vi "HandleServers.vi"(8 "error in (no error)":errorcluster, 11 "S4GUI in":refnum<class "S4GUI.lvclass">) -> (0 "error out":errorcluster, 3 "S4GUI out":refnum<class "S4GUI.lvclass">)   [LabVIEW 2018, in "S4GUI.lvclass"]
uses:
  S4GUI.lvclass
  S4GUI.lvclass/S4GUI.ctl
  Server/Server.lvclass/Server.ctl
  SyncBox/Sync Box.lvclass
  C:/Users/devstaff/sparc4/s4gui/Versao ZeroMQ REQ-REP/SPARC4_GUI -v1.0.8 - reconhecimento do ACK do ACS/Server/Server.lvclass
  Instrument/Instrument.lvclass
  TCS/TCS.lvclass
  Acquisition/Acquisition.lvclass
  TelFocus/TelFocus.lvclass
  WeatherStation/WeatherStation.lvclass
  GSserver/GSserver.lvclass
  Server/Server.lvclass
panel:
  out "resto (0-3)":u32
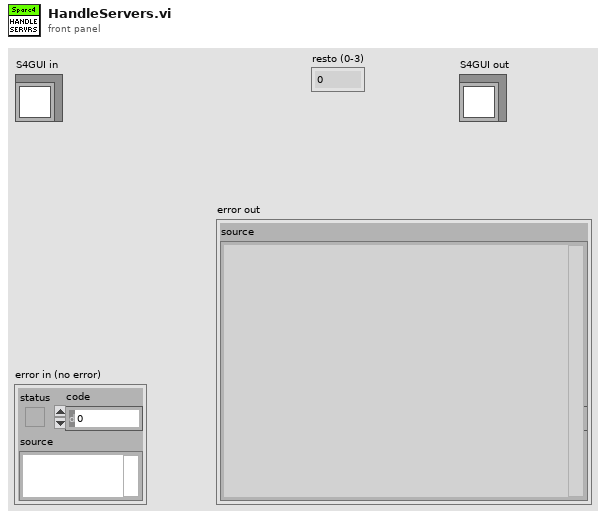
[diagram p1: front panel]
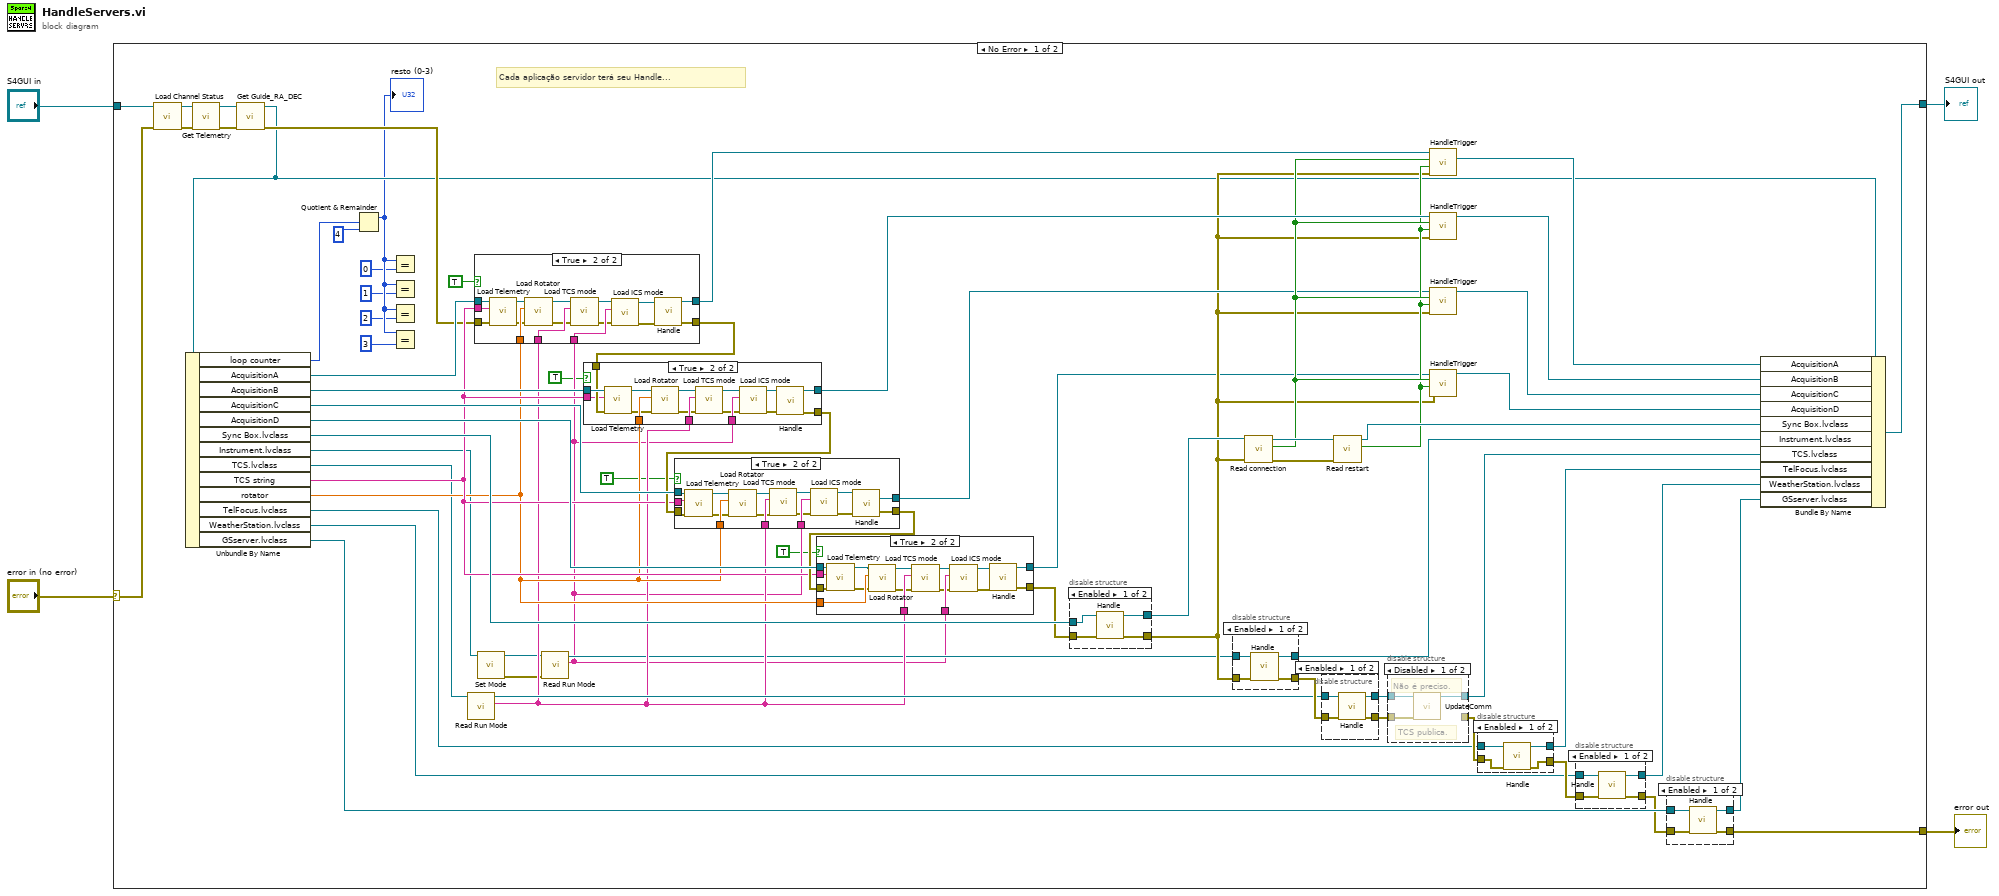
[diagram p0: block diagram]
diagram:
  n1 = case shown="No Error" "error in (no error)" {
    selector: "error in (no error)" -> [w14 w188]
    tunnel: [w5 w188] -> w3
    tunnel: [w73 w187] -> w1
    tunnel: "S4GUI in" -> [w12 w187]
    frame No Error {
      # "Cada aplicação servidor terá seu Handle..."
      n2 = call-dynamic "Load Channel Status.vi"("error in (no error)"=w14, "S4GUI in"=w12) -> ("error out"=w13:errorcluster, "S4GUI out"=w11:refnum<class "S4GUI.lvclass">)  [unwired: 8 in]
      n3 = call-dynamic "Get Telemetry.vi"("error in (no error)"=w13, "S4GUI in"=w11) -> ("error out"=w32:errorcluster, "S4GUI out"=w33:refnum<class "S4GUI.lvclass">)  [unwired: 8 in]
      n4 = call-dynamic "Get Guide_RA_DEC.vi"("error in (no error)"=w32, "S4GUI in"=w33) -> ("error out"=w31:errorcluster, "S4GUI out"=w30:refnum<class "S4GUI.lvclass">)  [unwired: 8 in]
      n5 = Unbundle By Name(w30) -> ("loop counter"=w10:u32, "AcquisitionA"=w61:refnum<class "Acquisition.lvclass">, "AcquisitionB"=w60:refnum<class "Acquisition.lvclass">, "AcquisitionC"=w58:refnum<class "Acquisition.lvclass">, "AcquisitionD"=w57:refnum<class "Acquisition.lvclass">, "Sync Box.lvclass"=w72:refnum<class "Sync Box.lvclass">, "Instrument.lvclass"=w39:refnum<class "Instrument.lvclass">, "TCS.lvclass"=w42:refnum<class "TCS.lvclass">, "TCS string"=w45:string, "rotator"=w43:dbl, "TelFocus.lvclass"=w18:refnum<class "TelFocus.lvclass">, "WeatherStation.lvclass"=w9:refnum<class "WeatherStation.lvclass">, "GSserver.lvclass"=w8:refnum<class "GSserver.lvclass">)
      n6 = Quotient & Remainder(x=w10, y=u32 4) -> (x-y*floor(x/y)=w28:u32)  [unwired: 1 out]
      "resto (0-3)" <- w28
      n7 = Equal?(x=w28, y=u32 0) -> ()  [unwired: 1 out]
      n8 = Equal?(x=w28, y=u32 1) -> ()  [unwired: 1 out]
      n9 = Equal?(x=w28, y=u32 2) -> ()  [unwired: 1 out]
      n10 = Equal?(x=w28, y=u32 3) -> ()  [unwired: 1 out]
      n11 = call-dynamic "Read Run Mode.vi"("Server in"=w42) -> ("Run mode"=w40:string, "Server out"=w41:refnum<class "TCS.lvclass">)  [unwired: 8 in, 1 out]
      n12 = call-dynamic "Set Mode.vi"("Instrument in"=w39) -> ("error out"=w37:errorcluster, "Instrument out"=w38:refnum<class "Instrument.lvclass">)  [unwired: 9 in]
      n13 = call-dynamic "Read Run Mode.vi"("error in (no error)"=w37, "Server in"=w38) -> ("Run mode"=w35:string, "Server out"=w36:refnum<class "Instrument.lvclass">)  [unwired: 7 in, 1 out]
      n14 = case shown="True" TRUE {
        tunnel: [w159 w175] -> w67
        tunnel: w61 -> [w159 w174]
        tunnel: [w158 w173] -> w59
        tunnel: w45 -> [_ w172]
        tunnel: w43 -> [_ w171]
        tunnel: w40 -> [_ w170]
        tunnel: w35 -> [_ w169]
        tunnel: w31 -> [w158 w168]
        frame False {
        }
        frame True {
          n15 = call-dynamic "Load Telemetry.vi"("error in (no error)"=w168, "TCS telemetry"=w172, "Acquisition in"=w174) -> ("error out"=w166:errorcluster, "Acquisition out"=w167:refnum<class "Acquisition.lvclass">)  [unwired: 7 in]
          n16 = call-dynamic "Load Rotator.vi"("error in (no error)"=w166, "Rotator"=w171, "Acquisition in"=w167) -> ("error out"=w164:errorcluster, "Acquisition out"=w165:refnum<class "Acquisition.lvclass">)  [unwired: 7 in]
          n17 = call-dynamic "Load TCS mode.vi"("error in (no error)"=w164, "tcs mode"=w170, "Acquisition in"=w165) -> ("error out"=w161:errorcluster, "Acquisition out"=w163:refnum<class "Acquisition.lvclass">)  [unwired: 7 in]
          n18 = call-dynamic "Load ICS mode.vi"("error in (no error)"=w161, "ICS mode"=w169, "Acquisition in"=w163) -> ("error out"=w160:errorcluster, "Acquisition out"=w162:refnum<class "Acquisition.lvclass">)  [unwired: 7 in]
          n19 = call-dynamic "Handle.vi"("error in (no error)"=w160, "Acquisition in"=w162) -> ("error out"=w173:errorcluster, "Acquisition out"=w175:refnum<class "Acquisition.lvclass">)  [unwired: 8 in]
        }
      }
      n20 = case shown="True" TRUE {
        tunnel: [w141 w157] -> w68
        tunnel: w60 -> [w141 w156]
        tunnel: w59 -> [w140 w155]
        tunnel: [w140 w154] -> w56
        tunnel: w45 -> [_ w153]
        tunnel: w43 -> [_ w152]
        tunnel: w40 -> [_ w151]
        tunnel: w35 -> [_ w150]
        frame False {
        }
        frame True {
          n21 = call-dynamic "Load Telemetry.vi"("error in (no error)"=w155, "TCS telemetry"=w153, "Acquisition in"=w156) -> ("error out"=w148:errorcluster, "Acquisition out"=w149:refnum<class "Acquisition.lvclass">)  [unwired: 7 in]
          n22 = call-dynamic "Load Rotator.vi"("error in (no error)"=w148, "Rotator"=w152, "Acquisition in"=w149) -> ("error out"=w146:errorcluster, "Acquisition out"=w147:refnum<class "Acquisition.lvclass">)  [unwired: 7 in]
          n23 = call-dynamic "Load TCS mode.vi"("error in (no error)"=w146, "tcs mode"=w151, "Acquisition in"=w147) -> ("error out"=w143:errorcluster, "Acquisition out"=w145:refnum<class "Acquisition.lvclass">)  [unwired: 7 in]
          n24 = call-dynamic "Load ICS mode.vi"("error in (no error)"=w143, "ICS mode"=w150, "Acquisition in"=w145) -> ("error out"=w142:errorcluster, "Acquisition out"=w144:refnum<class "Acquisition.lvclass">)  [unwired: 7 in]
          n25 = call-dynamic "Handle.vi"("error in (no error)"=w142, "Acquisition in"=w144) -> ("error out"=w154:errorcluster, "Acquisition out"=w157:refnum<class "Acquisition.lvclass">)  [unwired: 8 in]
        }
      }
      n26 = case shown="True" TRUE {
        tunnel: w58 -> [w123 w139]
        tunnel: w56 -> [w122 w138]
        tunnel: [w122 w137] -> w55
        tunnel: [w123 w136] -> w47
        tunnel: w45 -> [_ w135]
        tunnel: w43 -> [_ w134]
        tunnel: w40 -> [_ w133]
        tunnel: w35 -> [_ w132]
        frame False {
        }
        frame True {
          n27 = call-dynamic "Load Telemetry.vi"("error in (no error)"=w138, "TCS telemetry"=w135, "Acquisition in"=w139) -> ("error out"=w130:errorcluster, "Acquisition out"=w131:refnum<class "Acquisition.lvclass">)  [unwired: 7 in]
          n28 = call-dynamic "Load Rotator.vi"("error in (no error)"=w130, "Rotator"=w134, "Acquisition in"=w131) -> ("error out"=w129:errorcluster, "Acquisition out"=w128:refnum<class "Acquisition.lvclass">)  [unwired: 7 in]
          n29 = call-dynamic "Load TCS mode.vi"("error in (no error)"=w129, "tcs mode"=w133, "Acquisition in"=w128) -> ("error out"=w127:errorcluster, "Acquisition out"=w126:refnum<class "Acquisition.lvclass">)  [unwired: 7 in]
          n30 = call-dynamic "Load ICS mode.vi"("error in (no error)"=w127, "ICS mode"=w132, "Acquisition in"=w126) -> ("error out"=w125:errorcluster, "Acquisition out"=w124:refnum<class "Acquisition.lvclass">)  [unwired: 7 in]
          n31 = call-dynamic "Handle.vi"("error in (no error)"=w125, "Acquisition in"=w124) -> ("error out"=w137:errorcluster, "Acquisition out"=w136:refnum<class "Acquisition.lvclass">)  [unwired: 8 in]
        }
      }
      n32 = case shown="True" TRUE {
        tunnel: [w104 w121] -> w71
        tunnel: w57 -> [w105 w120]
        tunnel: w55 -> [w104 w119]
        tunnel: w45 -> [_ w118]
        tunnel: w43 -> [_ w117]
        tunnel: w40 -> [_ w116]
        tunnel: w35 -> [_ w115]
        tunnel: [w105 w114] -> w34
        frame False {
        }
        frame True {
          n33 = call-dynamic "Load Telemetry.vi"("error in (no error)"=w119, "TCS telemetry"=w118, "Acquisition in"=w120) -> ("error out"=w112:errorcluster, "Acquisition out"=w113:refnum<class "Acquisition.lvclass">)  [unwired: 7 in]
          n34 = call-dynamic "Load Rotator.vi"("error in (no error)"=w112, "Rotator"=w117, "Acquisition in"=w113) -> ("error out"=w111:errorcluster, "Acquisition out"=w110:refnum<class "Acquisition.lvclass">)  [unwired: 7 in]
          n35 = call-dynamic "Load TCS mode.vi"("error in (no error)"=w111, "tcs mode"=w116, "Acquisition in"=w110) -> ("error out"=w108:errorcluster, "Acquisition out"=w109:refnum<class "Acquisition.lvclass">)  [unwired: 7 in]
          n36 = call-dynamic "Load ICS mode.vi"("error in (no error)"=w108, "ICS mode"=w115, "Acquisition in"=w109) -> ("error out"=w107:errorcluster, "Acquisition out"=w106:refnum<class "Acquisition.lvclass">)  [unwired: 7 in]
          n37 = call-dynamic "Handle.vi"("error in (no error)"=w107, "Acquisition in"=w106) -> ("error out"=w121:errorcluster, "Acquisition out"=w114:refnum<class "Acquisition.lvclass">)  [unwired: 8 in]
        }
      }
      n38 = disable-structure shown="Enabled" {
        disable-tunnel: [w184 w185] -> w46
        disable-tunnel: w72 -> [w183 w186]
        disable-tunnel: [w182 w186] -> w48
        disable-tunnel: w71 -> [w181 w185]
        frame Enabled {
          n39 = call-dynamic "Handle.vi"("error in (no error)"=w181, "Sync Box in"=w183) -> ("error out"=w184:errorcluster, "Sync Box out"=w182:refnum<class "Sync Box.lvclass">)  [unwired: 8 in]
        }
        frame Disabled {
        }
      }
      n40 = disable-structure shown="Enabled" {
        disable-tunnel: [w95 w97] -> w70
        disable-tunnel: w46 -> [w94 w96]
        disable-tunnel: [w93 w96] -> w44
        disable-tunnel: w36 -> [w92 w97]
        frame Enabled {
          n41 = call-dynamic "Handle.vi"("error in (no error)"=w94, "Instrument in"=w92) -> ("error out"=w93:errorcluster, "Instrument out"=w95:refnum<class "Instrument.lvclass">)  [unwired: 8 in]
        }
        frame Disabled {
        }
      }
      n42 = call "Read connection.vi"("error in (no error)"=w46, "Server in"=w48) -> ("error out"=w51:errorcluster, "connection"=w50:bool, "Server out"=w52:refnum<class "Sync Box.lvclass">)  [unwired: 7 in]
      n43 = disable-structure shown="Enabled" {
        disable-tunnel: [w89 w90] -> w54
        disable-tunnel: [w88 w91] -> w53
        disable-tunnel: w44 -> [w87 w90]
        disable-tunnel: w41 -> [w86 w91]
        frame Enabled {
          n44 = call-dynamic "Handle.vi"("error in (no error)"=w87, "TCS in"=w86) -> ("error out"=w89:errorcluster, "TCS out"=w88:refnum<class "TCS.lvclass">)  [unwired: 8 in]
        }
        frame Disabled {
        }
      }
      n45 = call-dynamic "Read restart.vi"("error in (no error)"=w51, "Server in"=w52) -> ("restart"=w49:bool, "Server out"=w69:refnum<class "Sync Box.lvclass">)  [unwired: 7 in, 1 out]
      n46 = disable-structure shown="Disabled" {
        disable-tunnel: [w178 w180] -> w62
        disable-tunnel: w54 -> [w177 w179]
        disable-tunnel: w53 -> [w176 w180]
        disable-tunnel: [_ w179] -> w19
        frame Disabled {
          # "TCS publica."
          # "Não é preciso."
          n47 = call-dynamic "UpdateComm.vi"("error in (no error)"=w177, "TCS in"=w176) -> ("TCS out"=w178:refnum<class "TCS.lvclass">)  [unwired: 8 in, 1 out]
        }
        frame Enabled {
        }
      }
      n48 = call-dynamic "HandleTrigger.vi"("error in (no error)"=w46, "SyncBox transition"=w49, "SyncBox status"=w50, "Acquisition in"=w67) -> ("Acquisition out"=w66:refnum<class "Acquisition.lvclass">)  [unwired: 6 in, 1 out]
      n49 = call-dynamic "HandleTrigger.vi"("error in (no error)"=w46, "SyncBox transition"=w49, "SyncBox status"=w50, "Acquisition in"=w68) -> ("Acquisition out"=w65:refnum<class "Acquisition.lvclass">)  [unwired: 6 in, 1 out]
      n50 = call-dynamic "HandleTrigger.vi"("error in (no error)"=w46, "SyncBox transition"=w49, "SyncBox status"=w50, "Acquisition in"=w47) -> ("Acquisition out"=w64:refnum<class "Acquisition.lvclass">)  [unwired: 6 in, 1 out]
      n51 = call-dynamic "HandleTrigger.vi"("error in (no error)"=w46, "SyncBox transition"=w49, "SyncBox status"=w50, "Acquisition in"=w34) -> ("Acquisition out"=w63:refnum<class "Acquisition.lvclass">)  [unwired: 6 in, 1 out]
      n52 = disable-structure shown="Enabled" {
        disable-tunnel: w19 -> [w101 w102]
        disable-tunnel: w18 -> [w100 w103]
        disable-tunnel: [w99 w103] -> w17
        disable-tunnel: [w98 w102] -> w16
        frame Enabled {
          n53 = call-dynamic "Handle.vi"("error in (no error)"=w101, "TelFocus in"=w100) -> ("error out"=w98:errorcluster, "TelFocus out"=w99:refnum<class "TelFocus.lvclass">)  [unwired: 8 in]
        }
        frame Disabled {
        }
      }
      n54 = disable-structure shown="Enabled" {
        disable-tunnel: w16 -> [w83 w84]
        disable-tunnel: [w82 w85] -> w15
        disable-tunnel: w9 -> [w81 w85]
        disable-tunnel: [w80 w84] -> w6
        frame Enabled {
          n55 = call-dynamic "Handle.vi"("error in (no error)"=w83, "WeatherStation in"=w81) -> ("error out"=w80:errorcluster, "WeatherStation out"=w82:refnum<class "WeatherStation.lvclass">)  [unwired: 8 in]
        }
        frame Disabled {
        }
      }
      n56 = disable-structure shown="Enabled" {
        disable-tunnel: w8 -> [w77 w79]
        disable-tunnel: [w76 w79] -> w7
        disable-tunnel: w6 -> [w75 w78]
        disable-tunnel: [w74 w78] -> w5
        frame Enabled {
          n57 = call-dynamic "Handle.vi"("error in (no error)"=w75, "GSserver in"=w77) -> ("error out"=w74:errorcluster, "GSserver out"=w76:refnum<class "GSserver.lvclass">)  [unwired: 8 in]
        }
        frame Disabled {
        }
      }
      n58 = Bundle By Name(cluster=w30, "AcquisitionA"=w66, "AcquisitionB"=w65, "AcquisitionC"=w64, "AcquisitionD"=w63, "Sync Box.lvclass"=w69, "Instrument.lvclass"=w70, "TCS.lvclass"=w62, "TelFocus.lvclass"=w17, "WeatherStation.lvclass"=w15, "GSserver.lvclass"=w7) -> (w73:refnum<class "S4GUI.lvclass">)
    }
    frame Error {
    }
  }
  "error out" <- w3
  "S4GUI out" <- w1
